vi "Controller LNLS Control BPM Communication Loop.vi"(7 "Sync Objects":T1, 8 "error in (no error)":errorcluster, 11 "FOFB Configuration":T4={"FOFB Parameters"={"Network"={"FOFB Controller IP"="", "LNLS Control Network IP"="", "LNLS Control Network Power Supplies TCP Port"=0, "LNLS Control Network FOFB Configuration TCP Port"=0, "LNLS Control Network BPMs TCP Port"=0, "Monitoring Data TCP Port"=0, "Fast Archiver TCP Port"=0, "Fast Command TCP Port"=0, "TCP Listening Timeout"=0}, "Fast Acquisition"={"Sampling Period"=0, "Data Buffer Size"=0, "Monitoring Period"=0}, "Acquisition Network"=[], "Actuation Network"=[]}, "Number of Acquisition Chassis"=0, "Number of Actuation Chassis"=0, "Number of BPM Readings"=0, "BPM Reading Names"=[], "Selected BPM Readings"=[0, 1, 2, 3, 4, 5, 6, 7, 8, 9, 10, 11, 12, 13, 14, 15, 16, 17, 18, 19, 20, 21, 22, 23, 24, 25, 26, 27, 28, 29, 30, 31, 32, 33, 34, 35, 36, 37, 38, 39, 40, 41, 42, 43, 44, 45, 46, 47, 48, 49], "Number of Correctors"=0, "Corrector Names"=[], "Selected Correctors"=[0, 1, 2, 3, 4, 5, 6, 7, 8, 9, 10, 11, 12, 13, 14, 15, 16, 17, 18, 19, 20, 21, 22, 23, 24, 25, 26, 27, 28, 29, 30, 31, 32, 33, 34, 35, 36, 37, 38, 39, 40, 41, 42, 43, 44, 45, 46, 47, 48, 49], "Response Matrix"=[], "Reference Orbit"=[], "Correction Matrix"=[], "FPGA Filter Sets"=[], "Acquisition Chassis Names"=[], "Actuation Chassis Names"=[], "Acquisition Variables"=[], "Actuation Variables"=[], "PS Matrix Mapping"=[], "Inverse PS Matrix Mapping"=[], "BPM Matrix Mapping"=[], "Inverse BPM Matrix Mapping"=[], "BPM Planes"=[], "Corrector Planes"=[]}) -> (0 "error out":errorcluster)   [LabVIEW 2011, in "Controller Global Variables.lvlib"]
uses:
  Controller Global Variables.lvlib
  Types Definitions/Type FOFB Configuration.ctl
  Types Definitions/Type FOFB Parameters.ctl
  Types Definitions/Type Network Configuration.ctl
  Types Definitions/Type FA Configuration.ctl
  Types Definitions/Type Acquisition Network Configuration.ctl
  Types Definitions/Type Actuation Network Configuration.ctl
  Types Definitions/Type Synchronization Objects.ctl
  Types Definitions/Type Blocking Synchronization Objects.ctl
  Types Definitions/Type Monitoring Data.ctl
  Types Definitions/Type Operation Mode State.ctl
  Types Definitions/Type Diagnostics Data.ctl
  Types Definitions/Type CPU Loads Array.ctl
  Types Definitions/Type CPU Loads.ctl
  Types Definitions/Type Non-blocking Synchronization Objects.ctl
  Types Definitions/Type FOFB Variables.ctl
  Types Definitions/Type Actuation State.ctl
  Types Definitions/Type TCP State.ctl
  <vilib>/Platform/TimedLoop/XDataNode/timing_clust.ctl
  <vilib>/Platform/TimedLoop/XDataNode/nitl_modes.ctl
  <vilib>/Platform/TimedLoop/XDataNode/wakeup.ctl
  Controller Global Variables/Monitoring Data.vi
  LNLS Control VIs/LNLS Control Saturation minus10 10.vi
  <vilib>/Platform/TimedLoop/XDataNode/XDataNode.xnode
  Type Definitions.lvlib
  LNLS Control VIs.lvlib
  Misc VIs.lvlib
  <vilib>/Platform/TimedLoop/XDataNode/XDNodeRunTimeDep.lvlib
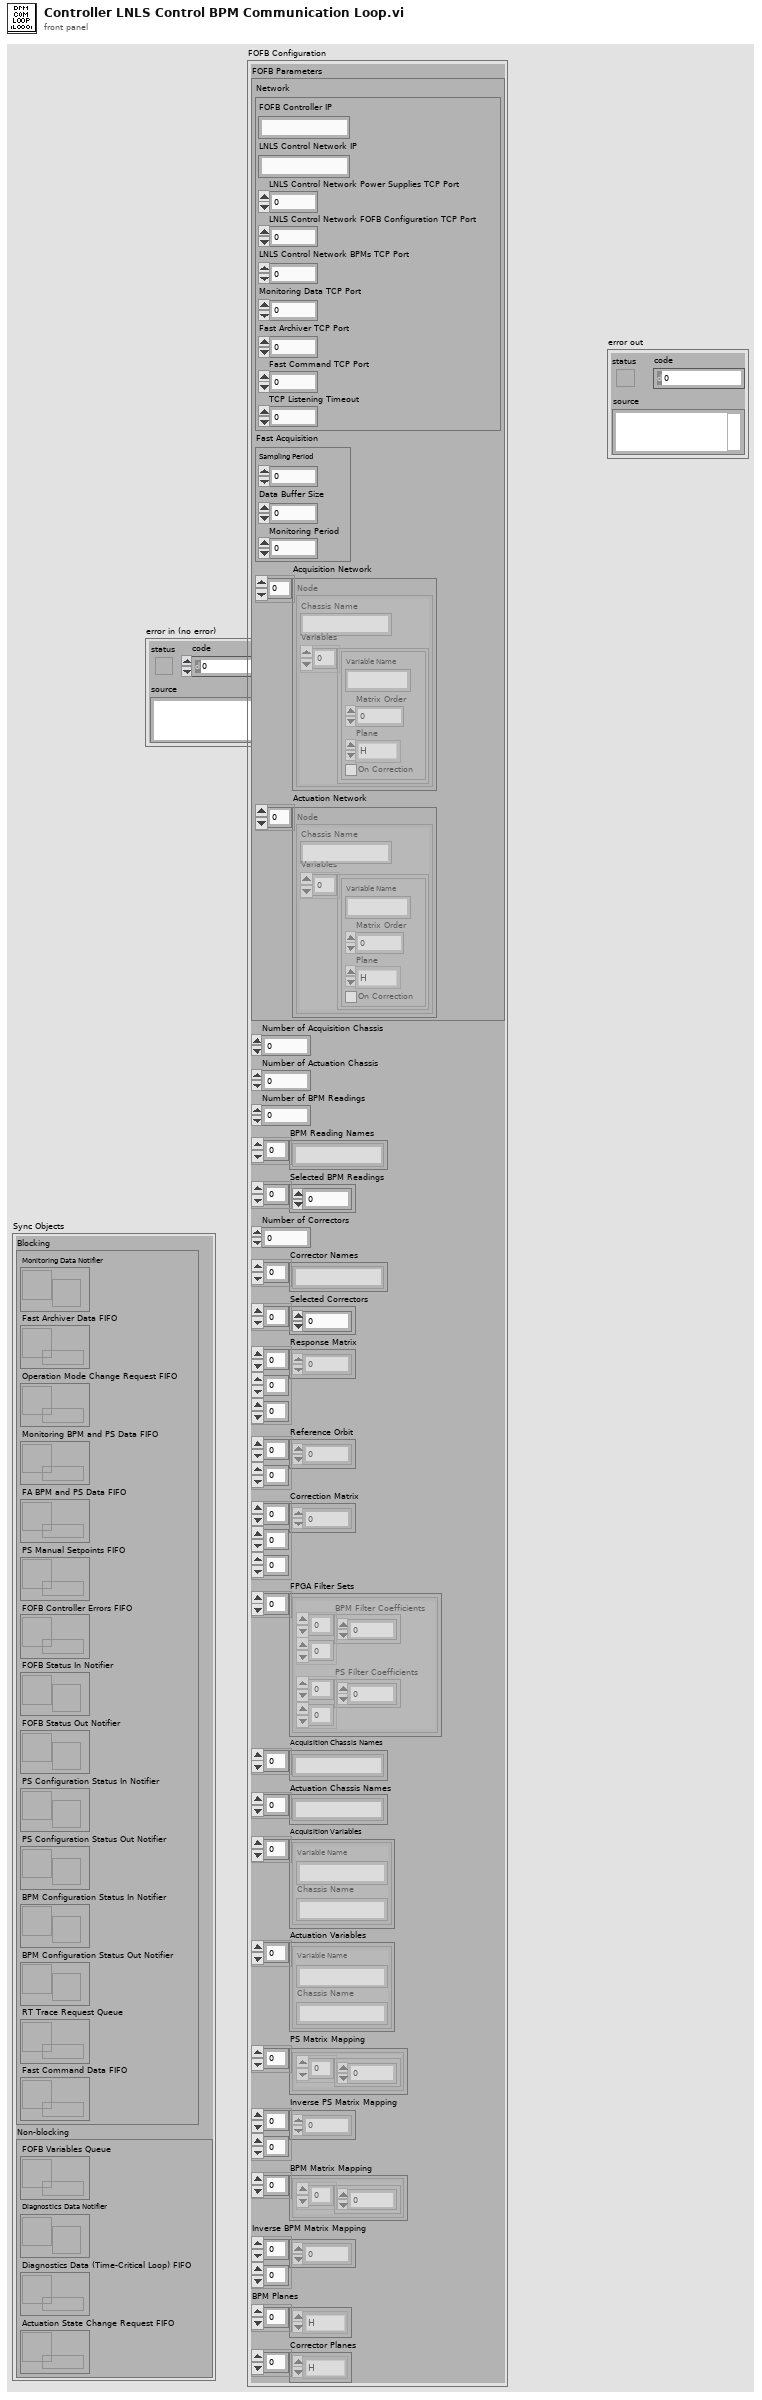
[diagram p1: front panel]
types:
  T1 = typedef "Type Definitions.lvlib/Type Synchronization Objects.ctl" = cluster{"Blocking":T2, "Non-blocking":T3}
  T2 = typedef "Type Definitions.lvlib/Type Blocking Synchronization Objects.ctl" = cluster{"Monitoring Data Notifier":refnum<notifier>, "Fast Archiver Data FIFO":refnum<queue>, "Operation Mode Change Request FIFO":refnum<k33>, "Monitoring BPM and PS Data FIFO":refnum<k33>, "FA BPM and PS Data FIFO":refnum<k33>, "PS Manual Setpoints FIFO":refnum<k33>, "FOFB Controller Errors FIFO ":refnum<k33>, "FOFB Status In Notifier":refnum<notifier>, "FOFB Status Out Notifier":refnum<notifier>, "PS Configuration Status In Notifier":refnum<notifier>, "PS Configuration Status Out Notifier":refnum<notifier>, "BPM Configuration Status In Notifier":refnum<notifier>, "BPM Configuration Status Out Notifier":refnum<notifier>, "RT Trace Request Queue":refnum<queue>, "Fast Command Data FIFO":refnum<k33>}
  T3 = typedef "Type Definitions.lvlib/Type Non-blocking Synchronization Objects.ctl" = cluster{"FOFB Variables Queue":refnum<queue>, "Diagnostics Data Notifier":refnum<notifier>, "Diagnostics Data (Time-Critical Loop) FIFO":refnum<k33>, "Actuation State Change Request FIFO":refnum<k33>}
  T4 = typedef "Type Definitions.lvlib/Type FOFB Configuration.ctl" = cluster{"FOFB Parameters":T5, "Number of Acquisition Chassis":i32, "Number of Actuation Chassis":i32, "Number of BPM Readings":i32, "BPM Reading Names":string[], "Selected BPM Readings":u32[], "Number of Correctors":i32, "Corrector Names":string[], "Selected Correctors":u32[], "Response Matrix":dbl[][][], "Reference Orbit":dbl[][], "Correction Matrix":dbl[][][], "FPGA Filter Sets":cluster{"BPM Filter Coefficients":dbl[][], "PS Filter Coefficients":dbl[][]}[], "Acquisition Chassis Names":string[], "Actuation Chassis Names":string[], "Acquisition Variables":cluster{"Variable Name":string, "Chassis Name":string}[], "Actuation Variables":cluster{"Variable Name":string, "Chassis Name":string}[], "PS Matrix Mapping":cluster{u32[]}[], "Inverse PS Matrix Mapping":u32[][], "BPM Matrix Mapping":cluster{u32[]}[], "Inverse BPM Matrix Mapping":u32[][], "BPM Planes":enum8{"H", "V"}[], "Corrector Planes":enum8{"H", "V"}[]}
  T5 = typedef "Type Definitions.lvlib/Type FOFB Parameters.ctl" = cluster{"Network":T6, "Fast Acquisition":T7, "Acquisition Network":T8, "Actuation Network":T9}
  T6 = typedef "Type Definitions.lvlib/Type Network Configuration.ctl" = cluster{"FOFB Controller IP":string, "LNLS Control Network IP":string, "LNLS Control Network Power Supplies TCP Port":u16, "LNLS Control Network FOFB Configuration TCP Port":u16, "LNLS Control Network BPMs TCP Port":u16, "Monitoring Data TCP Port":u16, "Fast Archiver TCP Port":u16, "Fast Command TCP Port":u16, "TCP Listening Timeout":i32}
  T7 = typedef "Type Definitions.lvlib/Type FA Configuration.ctl" = cluster{"Sampling Period":u32, "Data Buffer Size":u32, "Monitoring Period":u32}
  T8 = typedef "Type Definitions.lvlib/Type Acquisition Network Configuration.ctl" = cluster{"Chassis Name":string, "Variables":cluster{"Variable Name":string, "Matrix Order":u32, "Plane":enum8{"H", "V"}, "On Correction":bool}[]}[]
  T9 = typedef "Type Definitions.lvlib/Type Actuation Network Configuration.ctl" = cluster{"Chassis Name":string, "Variables":cluster{"Variable Name":string, "Matrix Order":u32, "Plane":enum8{"H", "V"}, "On Correction":bool}[]}[]
  T10 = typedef "Type Definitions.lvlib/Type TCP State.ctl" = enum16{"Idle", "Wait Connection", "Read Data", "Process Data", "Write Data", "Close Connection"}
  T11 = typedef "XDNodeRunTimeDep.lvlib/timing_clust.ctl" = cluster{"Expected End [f-1]":u64, "Actual End [f-1]":u64, "Finished Late? [f-1]":bool, "Expected End [i-1]":u64, "Actual End [i-1]":u64, "Finished Late? [i-1]":bool, "Expected Start [i]":u64, "Actual Start [i]":u64, "Expected Start [f]":u64, "Actual Start [f]":u64, "Source Name":string, "Structure Name":string, "Period":i64, "Deadline":i64, "Offset":i64, "Start":i64, "Priority":i32, "Timeout":i32, "Mode":T12, "Wakeup Reason":T13, "Error":errorcluster, "Source Type":string, "Secondary Source Type":string, "Global End Time":u64, "Global Start Time":u64, "Frame Duration":u64, "Iteration Duration":u64, "Assigned CPU":i32, "I/O Scan Engine Mode":u32}
  T12 = typedef "XDNodeRunTimeDep.lvlib/nitl_modes.ctl" = enum32{"No Change", "Process missed periods, maintain original phase", "Discard missed periods, maintain original phase", "Process missed periods, ignore original phase", "Discard missed periods, ignore original phase"}
  T13 = typedef "XDNodeRunTimeDep.lvlib/wakeup.ctl" = enum32{"Normal", "Aborted", "Asynchronous wakeup", "Timing source error", "Timed loop error", "Timeout"}
  T14 = typedef "Type Definitions.lvlib/Type Monitoring Data.ctl" = cluster{"Timestamp":timestamp, "BPM Readings":dbl[], "PS Readings":dbl[], "PS FOFB Setpoints":dbl[], "PS Status per Rack":u8[], "PS ON-OFF per Rack":u8[], "Operation Mode":T15, "Diagnostics Data":T16, "Controller Status Table":i32[]}
  T15 = typedef "Type Definitions.lvlib/Type Operation Mode State.ctl" = enum8{"Idle Mode", "Manual Mode", "FOFB Mode"}
  T16 = typedef "Type Definitions.lvlib/Type Diagnostics Data.ctl" = cluster{"Time-Critical Loop Missed Iterations":u32, "Time-Critical Loop Execution Time (usec)":u32, "Available Memory (bytes)":u32, "CPU Loads Array":T17}
  T17 = typedef "Type Definitions.lvlib/Type CPU Loads Array.ctl" = T18[]
  T18 = typedef "Type Definitions.lvlib/Type CPU Loads.ctl" = cluster{"Total (%)":dbl, "Time Critical (%)":dbl, "Timed Structures (%)":dbl, "High (%)":dbl, "Above Normal (%)":dbl, "Normal (%)":dbl, "Background (%)":dbl, "Idle (%)":dbl, "ISR (%)":dbl}
  T19 = typedef "Type Definitions.lvlib/Type BPM Pre Encode.ctl" = cluster{"analog value":dbl, "status":u8}
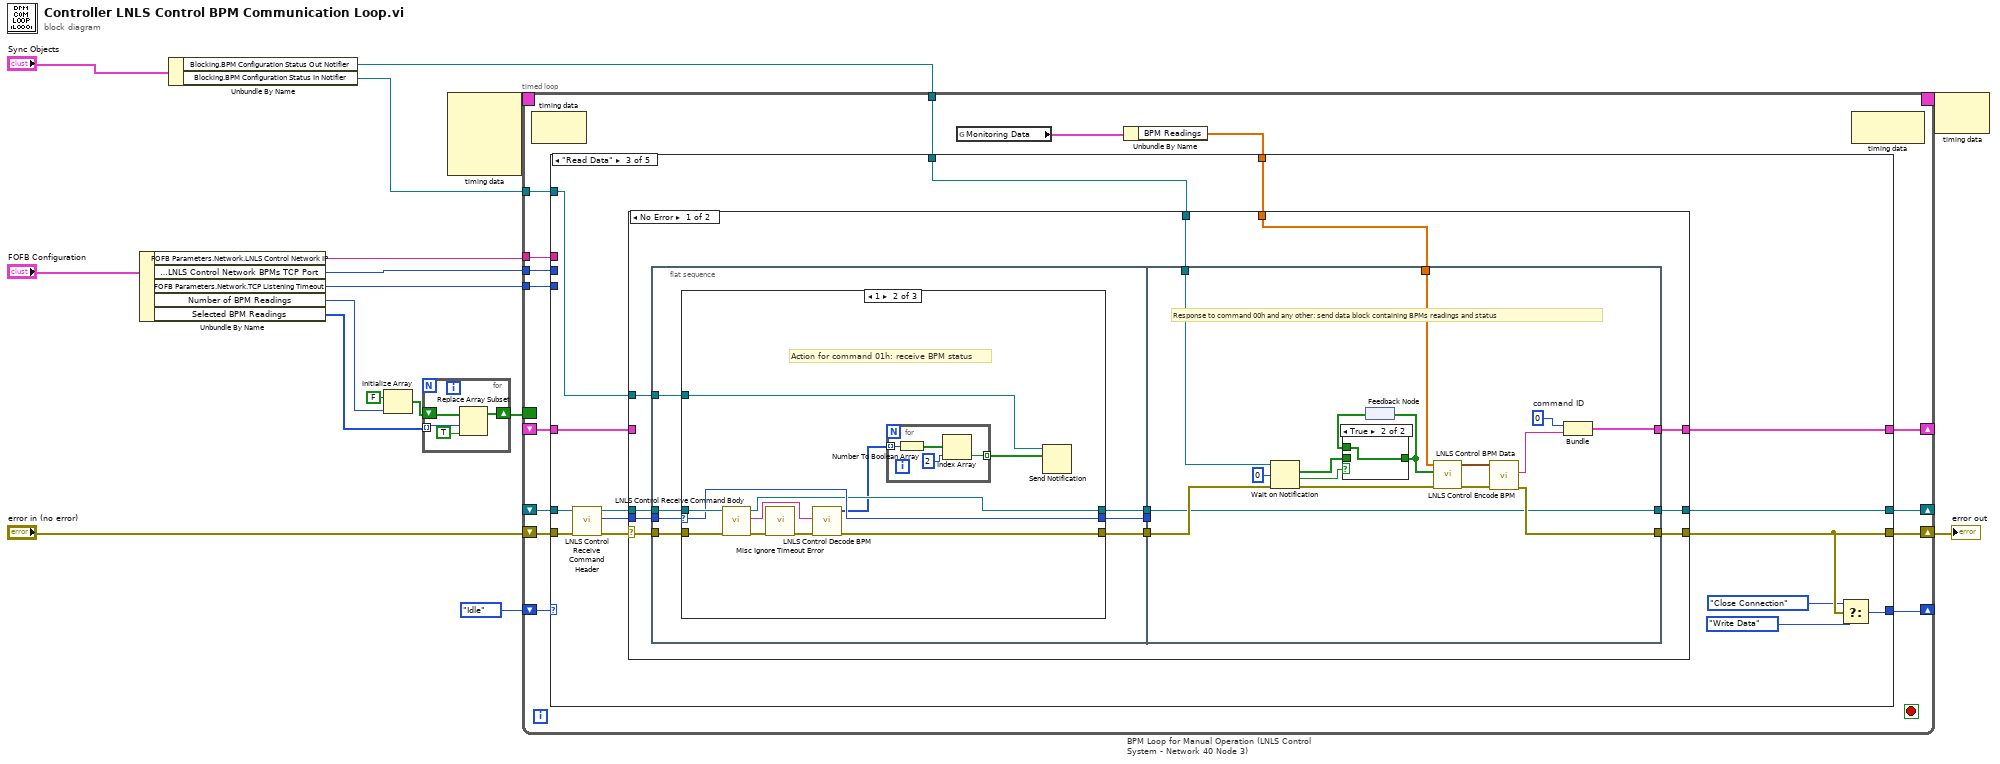
[diagram p0: block diagram]
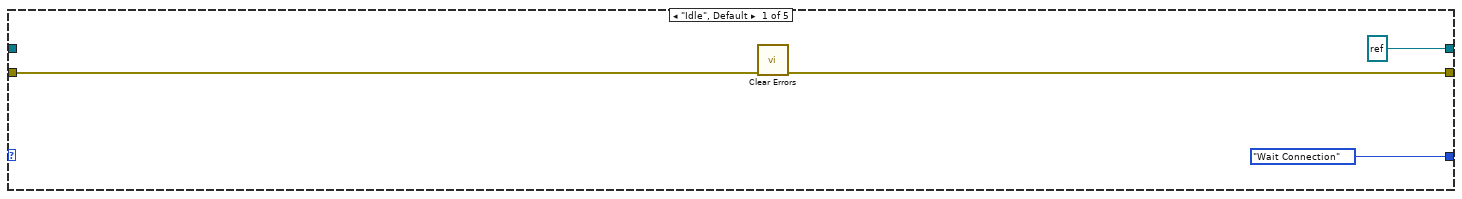
[diagram p2: hidden frame]
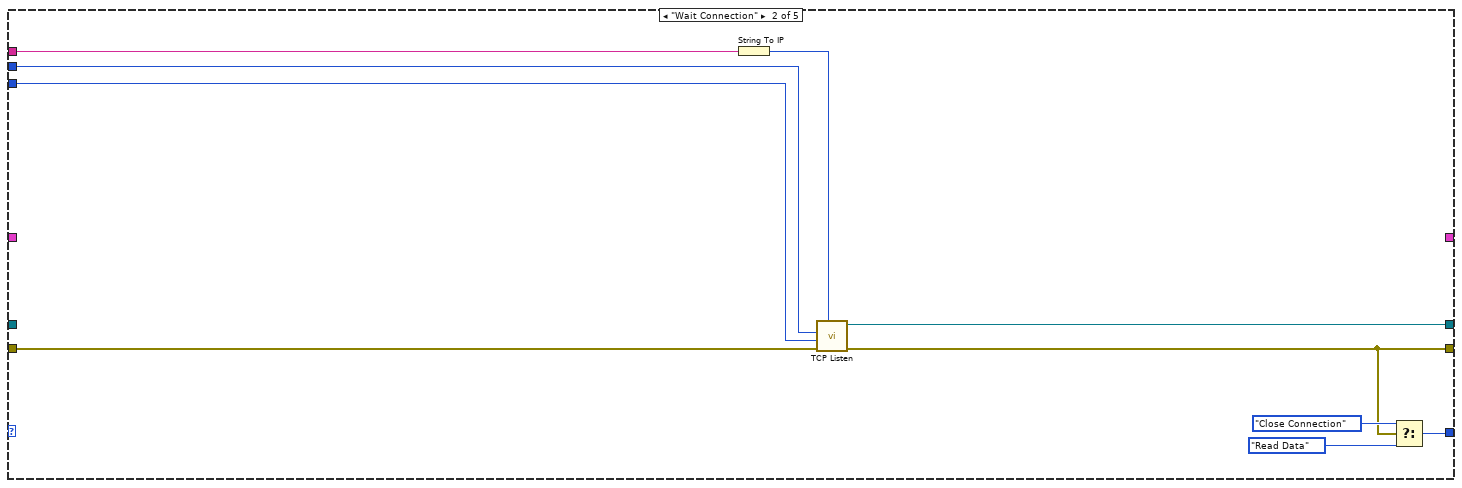
[diagram p3: hidden frame]
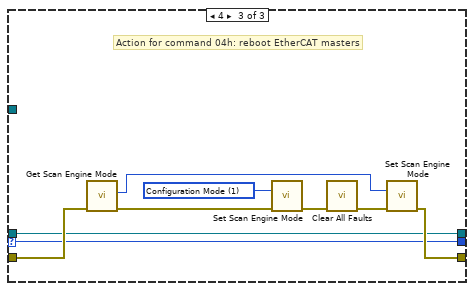
[diagram p5: hidden frame]
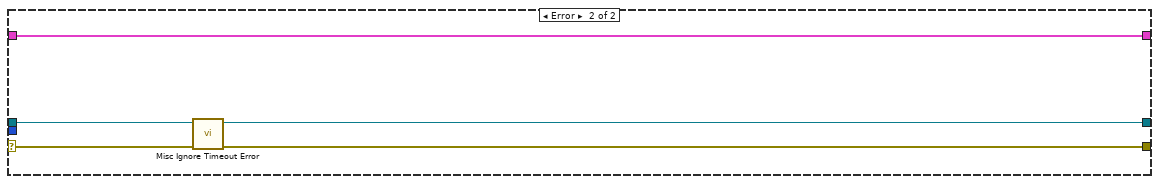
[diagram p7: hidden frame]
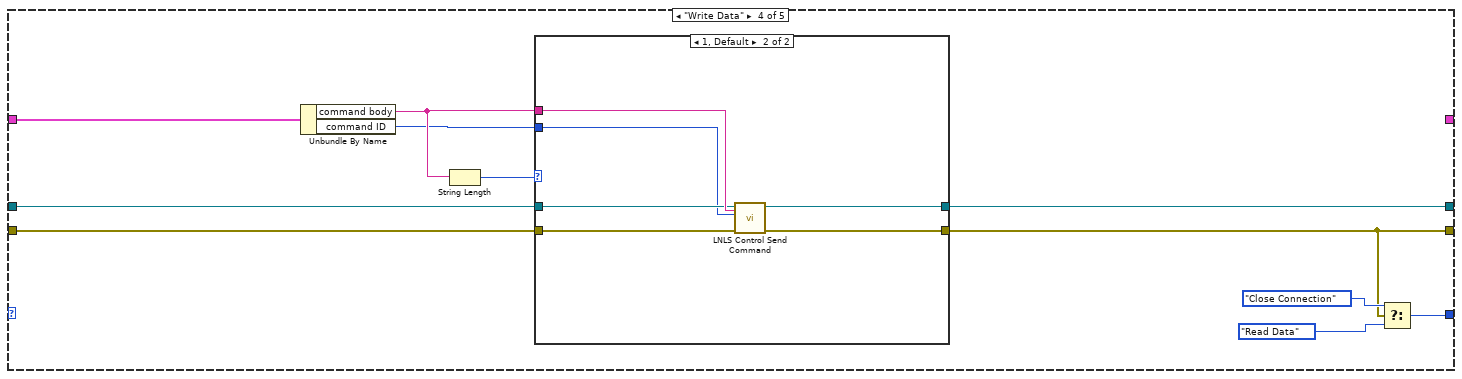
[diagram p8: hidden frame]
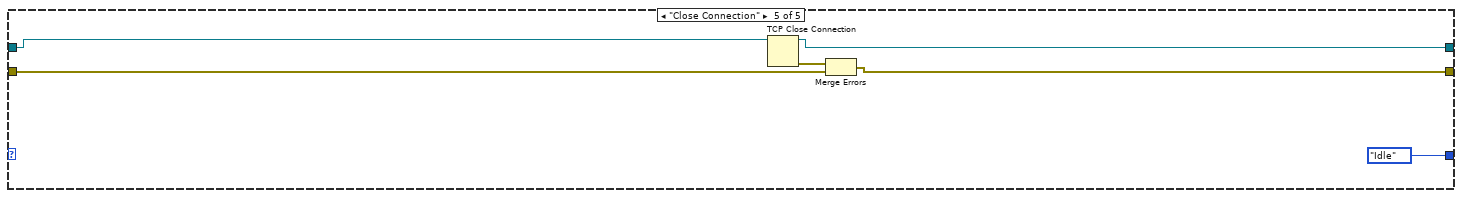
[diagram p10: hidden frame]
diagram:
  n1 = Unbundle By Name("FOFB Configuration") -> ("FOFB Parameters.Network.LNLS Control Network IP"=w10:string, "FOFB Parameters.Network.LNLS Control Network BPMs TCP Port"=w9:u16, "FOFB Parameters.Network.TCP Listening Timeout"=w8:i32, "Number of BPM Readings"=w3:i32, "Selected BPM Readings"=w2:u32[])
  n2 = Unbundle By Name("Sync Objects") -> ("Blocking.BPM Configuration Status Out Notifier"=w6:refnum<notifier>, "Blocking.BPM Configuration Status In Notifier"=w7:refnum<notifier>)
  n3 = Initialize Array(FALSE, w3) -> (w4:bool[])
  n4 = for {
    tunnel: w2 -> [w21] mode=indexing
    shift-right: [w18] -> w1
    shift-left: w4 -> [w20]
    n5 = Replace Array Subset(array=w20, new element=TRUE ("new element/subarray"), index=w21) -> (w18:bool[])
  }
  n6 = node-c288() -> (w17:T11)  [unwired: 4 in]
  n7 = timed-loop "BPM Loop for Manual Operation (LNLS Control System - Network 40 Node 3)" {
    shift-right: [w34] -> _
    shift-left: Type_TCP_State."Idle" ("f") -> [w36]
    shift-right: [w35] -> _
    shift-left: _ -> [w33]
    shift-right: [w22] -> w13
    shift-left: "error in (no error)" -> [w29]
    shift-right: [w31] -> _
    shift-left: _ -> [w30]
    tunnel: w9 -> [w32]
    tunnel: w10 -> [w28]
    tunnel: w8 -> [w27]
    timing: w17 -> [_]
    timing-out: [_] -> w16
    tunnel: w7 -> [w24]
    tunnel: w6 -> [w23]
    border: w1 -> [_]
    stop <- _ stop-if-true
    n8 = node-c288() -> ()  [unwired: 1 in, 1 out]
    n9 = global read "Monitoring Data.vi" "Monitoring Data"() -> (w26:T14)
    n10 = Unbundle By Name(w26) -> ("BPM Readings"=w25:dbl[])
    n11 = case shown="\"Read Data\"" w36 {
      tunnel: [refnum<k5> refnum ("connection ID") w49 w67 w139 w159] -> w35
      tunnel: [w40 w44 w65 w138 w155] -> w22
      tunnel: [Type_TCP_State."Wait Connection" w52 w66 w144 Type_TCP_State."Idle"] -> w34
      tunnel: w33 -> [_ _ w63 w141 w160]
      tunnel: w29 -> [w39 w45 w64 w140 w157]
      tunnel: w32 -> [_ w48 _ _ _]
      tunnel: [_ _ w60 _ _] -> w31
      tunnel: w30 -> [_ _ w58 w143 _]
      tunnel: w28 -> [_ w46 _ _ _]
      tunnel: w27 -> [_ w43 _ _ _]
      tunnel: w25 -> [_ _ w55 _ _]
      tunnel: w24 -> [_ _ w54 _ _]
      tunnel: w23 -> [_ _ w53 _ _]
      frame "Idle", Default {
        n12 = call <vilib>:"Clear Errors.vi"("error in (no error)"=w39) -> ("error out"=w40:errorcluster)  [unwired: 6 in]
      }
      frame "Wait Connection" {
        n13 = String To IP(1:w46) -> (0:w47:u32)
        n14 = call <vilib>:"TCP Listen.vi"("net address"=w47, "error in (no error)"=w45, "timeout ms (wait forever: -1)"=w43, "port"=w48) -> ("error out"=w44:errorcluster, "connection ID"=w49:refnum<k5>)  [unwired: 3 in, 3 out]
        n15 = Select(t=Type_TCP_State."Close Connection", s=w44, f=Type_TCP_State."Read Data") -> (s? t:f=w52:T10)
      }
      frame "Read Data" {
        n16 = call "LNLS Control Receive Command Header.vi"("error in (no error)"=w64, "connection ID"=w63) -> ("error out"=w59:errorcluster, "command ID"=w56:u8, "connection ID out"=w62:refnum<k5>)  [unwired: 7 in]
        n17 = case shown="No Error" w59 {
          selector: w59 -> [w74 w132]
          tunnel: [w79 w135] -> w67
          tunnel: [w78 w133] -> w65
          tunnel: w62 -> [w77 w135]
          tunnel: w56 -> [w76 _]
          tunnel: [w75 w134] -> w60
          tunnel: w58 -> [_ w134]
          tunnel: w55 -> [w70 _]
          tunnel: w54 -> [w69 _]
          tunnel: w53 -> [w68 _]
          frame No Error {
            n18 = flat-sequence {
              tunnel: [w86] -> w73
              tunnel: [w85] -> w72
              tunnel: w77 -> [w84]
              tunnel: w76 -> [w83]
              tunnel: w74 -> [w82]
              tunnel: [w81] -> w71
              tunnel: w69 -> [w80]
              tunnel: [w127] -> w79
              tunnel: w73 -> [w127]
              tunnel: [w129] -> w78
              tunnel: w72 -> [w128]
              tunnel: [w126] -> w75
              tunnel: w71 -> [_]
              tunnel: w70 -> [w120]
              tunnel: w68 -> [w125]
              frame #0 {
                n19 = case shown="1" w83 {
                  selector: w83 -> [w87 w98 w106]
                  tunnel: w82 -> [w89 w99 w113]
                  tunnel: [w89 w90 w112] -> w85
                  tunnel: [w88 w97 w105] -> w86
                  tunnel: w84 -> [w88 w100 w105]
                  tunnel: [w87 w98 w106] -> w81
                  tunnel: w80 -> [_ w91 _]
                  frame 0, Default {
                  }
                  frame 1 {
                    # "Action for command 01h: receive BPM status"
                    n20 = call "LNLS Control Receive Command Body.vi"("error in (no error)"=w99, "connection ID"=w100) -> ("error out"=w96:errorcluster, "command body"=w95:string, "connection ID out"=w97:refnum<k5>)  [unwired: 6 in, 1 out]
                    n21 = call "Misc Ignore Timeout Error.vi"("error in (no error)"=w96) -> ("error out"=w94:errorcluster)  [unwired: 9 in, 1 out]
                    n22 = call "LNLS Control Decode BPM.vi"("error in (no error)"=w94, "command body"=w95) -> ("error out"=w90:errorcluster, "BPM Control"=w92:u8[])  [unwired: 6 in]
                    n23 = for {
                      tunnel: w92 -> [w104] mode=indexing
                      tunnel: [w101] -> w93 mode=indexing
                      n24 = Number To Boolean Array(number=w104) -> (Boolean array=w103:bool[])
                      n25 = Index Array(array=w103, index=2) -> (element=w101:bool)
                    }
                    n26 = Send Notification(notification=w93, notifier=w91) -> ()  [unwired: 1 in, 2 out]
                  }
                  frame 4 {
                    w111 = 1 items=["Configuration Mode"=1, "Active Mode"=2] ("mode (Active Mode)")
                    # "Action for command 04h: reboot EtherCAT masters"
                    n27 = call <vilib>:"Get Scan Engine Mode.vi"("error in (no error)"=w113) -> ("error out"=w110:errorcluster, "mode"=w107:i32)  [unwired: 9 in]
                    n28 = call <vilib>:"Set Scan Engine Mode.vi"("mode (Active Mode)"=w111, "error in (no error)"=w110) -> ("error out"=w109:errorcluster)  [unwired: 13 in]
                    n29 = call <vilib>:"Clear All Faults.vi"("error in (no error)"=w109) -> ("error out"=w108:errorcluster)  [unwired: 1 in, 9 out]
                    n30 = call <vilib>:"Set Scan Engine Mode.vi"("mode (Active Mode)"=w107, "error in (no error)"=w108) -> ("error out"=w112:errorcluster)  [unwired: 13 in]
                  }
                }
              }
              frame #1 {
                w124 = u8 0  # command ID
                # "Response to command 00h and any other: send data block containing BPMs readings and status"
                n31 = Wait on Notification(notifier=w125, timeout in ms (-1)=0, error in (no error)=w128) -> (notification=w117:bool[], timed out?=w118:bool, error out=w121:errorcluster)  [unwired: 1 in, 1 out]
                n32 = feedback #1() -> (w115:bool[])
                n33 = case shown="True" w118 {
                  tunnel: w117 -> [w130 _]
                  tunnel: [w130 w131] -> w114
                  tunnel: w115 -> [_ w131]
                  frame False {
                  }
                  frame True {
                  }
                }
                n34 = feedback-in #1(w114) -> ()
                n35 = call "LNLS Control BPM Data.vi"("error in (no error)"=w121, "BPM Status (On correction?)"=w114, "BPM Readings"=w120) -> ("error out"=w123:errorcluster, "BPM Readings Data"=w119:T19[])  [unwired: 7 in]
                n36 = call "LNLS Control Encode BPM.vi"("error in (no error)"=w123, "BPM Data"=w119) -> ("error out"=w129:errorcluster, "command body"=w122:string)  [unwired: 8 in]
                n37 = Bundle("command ID"=w124, "command body"=w122) -> (w126:cluster{"command ID":u8, "command body":string})  [unwired: 1 in]
              }
            }
          }
          frame Error {
            n38 = call "Misc Ignore Timeout Error.vi"("error in (no error)"=w132) -> ("error out"=w133:errorcluster)  [unwired: 9 in, 1 out]
          }
        }
        n39 = Select(t=Type_TCP_State."Close Connection", s=w65, f=Type_TCP_State."Write Data") -> (s? t:f=w66:T10)
      }
      frame "Write Data" {
        n40 = Unbundle By Name(w143) -> ("command body"=w142:string, "command ID"=w137:u8)
        n41 = String Length(string=w142) -> (length=w136:i32)
        n42 = case shown="1, Default" w136 {
          tunnel: w142 -> [_ w154]
          tunnel: w141 -> [w148 w153]
          tunnel: w140 -> [w147 w152]
          tunnel: [w148 w151] -> w139
          tunnel: [w147 w150] -> w138
          tunnel: w137 -> [_ w149]
          frame 0 {
          }
          frame 1, Default {
            n43 = call "LNLS Control Send Command.vi"("command body"=w154, "error in (no error)"=w152, "command ID"=w149, "connection ID"=w153) -> ("error out"=w150:errorcluster, "connection ID out"=w151:refnum<k5>)  [unwired: 6 in]
          }
        }
        n44 = Select(t=Type_TCP_State."Close Connection", s=w138, f=Type_TCP_State."Read Data") -> (s? t:f=w144:T10)
      }
      frame "Close Connection" {
        n45 = TCP Close Connection(connection ID=w160) -> (connection ID out=w159:refnum<k5>, error out=w156:errorcluster)  [unwired: 2 in]
        n46 = Merge Errors(w156, w157) -> (w155:errorcluster)
      }
    }
    n47 = node-c288() -> ()  [unwired: 1 in, 1 out]
  }
  "error out" <- w13
  n48 = node-c288(w16) -> ()  [unwired: 1 out]
